vi "Is Null.vi"(8 "error in (no error)":errorcluster, 11 "Pointer in":refnum<class "Pointer.lvclass">) -> (0 "error out":errorcluster, 2 "null?":bool, 3 "Pointer out":refnum<class "Pointer.lvclass">)   [LabVIEW 2020, in "Memory Manager.lvlib" / "Pointer.lvclass"]
doc: "Checks if <b>Pointer</b> has an address of zero (null)."
uses:
  Pointer.lvclass
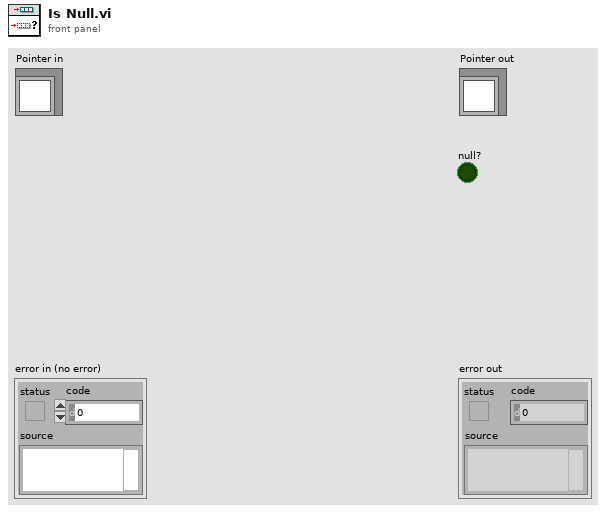
[diagram p1: front panel]
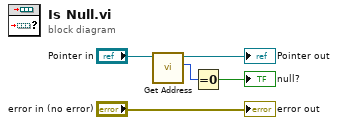
[diagram p0: block diagram]
diagram:
  n1 = call "Get Address.vi"("Pointer in"="Pointer in") -> ("address"=w2:u64, "Pointer out"=→"Pointer out":refnum<class "Pointer.lvclass">)  [unwired: 9 in]
  n2 = Equal To 0?(x=w2) -> (x = 0?=→"null?":bool)
  "error out" <- "error in (no error)"
